vi "System Settings.vi"(8 "Device Inputs":dbl[](array[numeric]), 10 "System Settings FIFO Indexes":T1, 11 "System Settings in":T2 {"HH Open Threshold [A]" min=0 max=8 format="%#_3p"; "HH ISeq Dur PS" items=["3.3ms @ 20MHz"=0, "6.5ms @ 10MHz"=4, "13ms @ 5MHz"=6, "26ms @ 2.5MHz"=7]; "HH Shoot Through Time [s]" min=0 max=0.003277 format="%#_3p"; "Clamp Fault Filter Time [s]" min=0 max=0.003277 format="%#_3p"; "DI HS Fault Filter Time [s]" min=0 max=0.003277 format="%#_3p"}) -> (3 "System Settings":T5 {"HH Open Threshold [A]" min=0 max=8 format="%#_3p"; "HH ISeq Dur PS" items=["3.3ms @ 20MHz"=0, "6.5ms @ 10MHz"=4, "13ms @ 5MHz"=6, "26ms @ 2.5MHz"=7]; "HH Shoot Through Time [s]" min=0 max=0.003277 format="%#_3p"; "Clamp Fault Filter Time [s]" min=0 max=0.003277 format="%#_3p"; "DI HS Fault Filter Time [s]" min=0 max=0.003277 format="%#_3p"})   [LabVIEW 2016, in "DCM Engine.lvlib"]
uses:
  DCM Engine.lvlib
  Built/DCM Classes Packed/Pharlap/C/DCM-Classes.lvlibp/DCM/Rev0/RT/System Settings.ctl
  Built/DCM Classes Packed/Pharlap/C/DCM-Classes.lvlibp/DCM/Rev0/RT/User LED.ctl
  Built/DCM Classes Packed/Pharlap/C/DCM-Classes.lvlibp/DCM/HH/RT/Duration Pre Scale.ctl
  <vilib>/Powertrain Controls/Device Drivers/DCM/Rev0/RT/System Settings.ctl
  <vilib>/Powertrain Controls/Device Drivers/DCM/Rev0/RT/User LED.ctl
  <vilib>/Powertrain Controls/Device Drivers/DCM/HH/RT/Duration Pre Scale.ctl
  Built/DCM Classes Packed/Pharlap/C/DCM-Classes.lvlibp/DCM/Rev0/RT/DCM - RT.lvclass
  Built/DCM Classes Packed/Pharlap/C/DCM-Classes.lvlibp/DCM/HH/RT/DCM - RT - HH.lvlib
  <vilib>/Powertrain Controls/Device Drivers/DCM/Rev0/RT/DCM - RT.lvclass
  <vilib>/Powertrain Controls/Device Drivers/DCM/HH/RT/DCM - RT - HH.lvlib
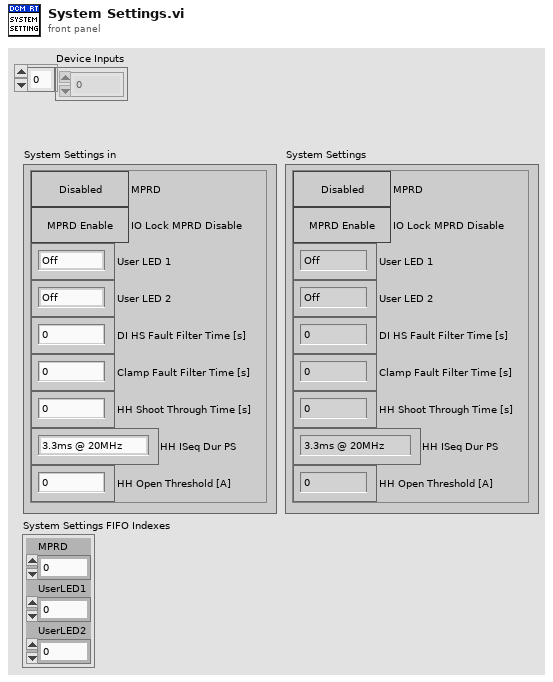
[diagram p1: front panel]
types:
  T1 = cluster{"MPRD":i32, "UserLED1":i32, "UserLED2":i32}
  T2 = typedef "DCM - RT.lvclass/System Settings.ctl" = cluster{"MPRD":bool, "IO Lock MPRD Disable":bool, "User LED 1":T3, "User LED 2":T3, "DI HS Fault Filter Time [s]":sgl, "Clamp Fault Filter Time [s]":sgl, "HH Shoot Through Time [s]":sgl, "HH ISeq Dur PS":T4, "HH Open Threshold [A]":sgl}
  T3 = typedef "DCM - RT.lvclass/User LED.ctl" = enum16{"Off", "Yellow", "Green"}
  T4 = typedef "DCM - RT - HH.lvlib/Duration Pre Scale.ctl" = u8
  T5 = typedef "DCM-Classes.lvlibp/DCM - RT.lvclass/System Settings.ctl" = cluster{"MPRD":bool, "IO Lock MPRD Disable":bool, "User LED 1":T6, "User LED 2":T6, "DI HS Fault Filter Time [s]":sgl, "Clamp Fault Filter Time [s]":sgl, "HH Shoot Through Time [s]":sgl, "HH ISeq Dur PS":T7, "HH Open Threshold [A]":sgl}
  T6 = typedef "DCM-Classes.lvlibp/DCM - RT.lvclass/User LED.ctl" = enum16{"Off", "Yellow", "Green"}
  T7 = typedef "DCM-Classes.lvlibp/DCM - RT - HH.lvlib/Duration Pre Scale.ctl" = u8
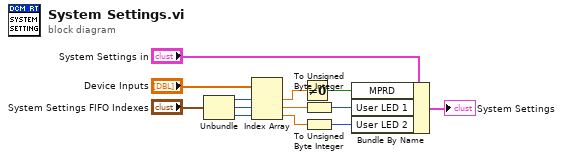
[diagram p0: block diagram]
diagram:
  n1 = Unbundle("System Settings FIFO Indexes") -> ("MPRD"=w10:i32, "UserLED1"=w12:i32, "UserLED2"=w11:i32)
  n2 = Index Array(array="Device Inputs", index #1=w10, index #2=w12, index #3=w11) -> (element #1=w8:dbl, element #2=w5:dbl, element #3=w6:dbl)
  n3 = Not Equal To 0?(x=w8) -> (x != 0?=w7:bool)
  n4 = To Unsigned Byte Integer(number=w5) -> (unsigned 8bit integer=w4:u8)
  n5 = To Unsigned Byte Integer(number=w6) -> (unsigned 8bit integer=w3:u8)
  n6 = Bundle By Name(cluster="System Settings in", "MPRD"=w7, "User LED 1"=w4, "User LED 2"=w3) -> (→"System Settings":T2)
